vi "PicoScopeospaAdvancedTriggerSettings.vi"(0 "handle in":i16=16384, 2 "Trigger holdoff (Samples)":u64, 5 "error in":errorcluster, 6 "Trigger Conditions":T7={"Channel A"=1, "Channel B"=0, "Channel C"=0, "Channel D"=0, "Channel E"=0, "Channel F"=0, "Channel G"=0, "Channel H"=0, "Port 0"=0, "Port 1"=0, "Aux"=0, "PWQ"=0, "Condition Logic"=0} {"Port 1" items=["Don't Care", "True", "False"]; "Channel H" items=["Don't Care", "True", "False"]; "Channel G" items=["Don't Care", "True", "False"]; "Channel F" items=["Don't Care", "True", "False"]; "Channel E" items=["Don't Care", "True", "False"]; "PWQ" items=["Don't Care", "True", "False"]; "Aux" items=["Don't Care", "True", "False"]; "Port 0" items=["Don't Care", "True", "False"]; "Channel D" items=["Don't Care", "True", "False"]; "Channel C" items=["Don't Care", "True", "False"]; "Channel B" items=["Don't Care", "True", "False"]; "Channel A" items=["Don't Care", "True", "False"]; "Condition Logic" items=["AND", "OR", "XOR"]}, 7 "Pulse Width Qualifier Conditions":T1 {"Port 1" items=["Don't Care", "True", "False"]; "Channel H" items=["Don't Care", "True", "False"]; "Channel G" items=["Don't Care", "True", "False"]; "Channel F" items=["Don't Care", "True", "False"]; "Channel E" items=["Don't Care", "True", "False"]; "Aux" items=["Don't Care", "True", "False"]; "Port 0" items=["Don't Care", "True", "False"]; "Channel D" items=["Don't Care", "True", "False"]; "Channel C" items=["Don't Care", "True", "False"]; "Channel B" items=["Don't Care", "True", "False"]; "Channel A" items=["Don't Care", "True", "False"]; "Condition Logic" items=["AND", "OR", "XOR"]}, 8 "Channel Trigger Properties":T5={"Channel A Trigger Properties"={"thresholdUpper"=0, "thresholdUpperHysteresis"=1638, "thresholdLower"=0, "thresholdLowerHysteresis"=1638, "Threshold Mode"=0, "Direction"=2, "Available"=TRUE}, "Channel B Trigger Properties"={"thresholdUpper"=0, "thresholdUpperHysteresis"=1638, "thresholdLower"=0, "thresholdLowerHysteresis"=1638, "Threshold Mode"=0, "Direction"=2, "Available"=FALSE}, "Channel C Trigger Properties"={"thresholdUpper"=0, "thresholdUpperHysteresis"=1638, "thresholdLower"=0, "thresholdLowerHysteresis"=1638, "Threshold Mode"=0, "Direction"=2, "Available"=FALSE}, "Channel D Trigger Properties"={"thresholdUpper"=0, "thresholdUpperHysteresis"=1638, "thresholdLower"=0, "thresholdLowerHysteresis"=1638, "Threshold Mode"=0, "Direction"=2, "Available"=FALSE}, "Channel E Trigger Properties"={"thresholdUpper"=0, "thresholdUpperHysteresis"=0, "thresholdLower"=0, "thresholdLowerHysteresis"=0, "Threshold Mode"=0, "Direction"=2, "Available"=FALSE}, "Channel F Trigger Properties"={"thresholdUpper"=0, "thresholdUpperHysteresis"=0, "thresholdLower"=0, "thresholdLowerHysteresis"=0, "Threshold Mode"=0, "Direction"=2, "Available"=FALSE}, "Channel G Trigger Properties"={"thresholdUpper"=0, "thresholdUpperHysteresis"=0, "thresholdLower"=0, "thresholdLowerHysteresis"=0, "Threshold Mode"=0, "Direction"=2, "Available"=FALSE}, "Channel H Trigger Properties"={"thresholdUpper"=0, "thresholdUpperHysteresis"=0, "thresholdLower"=0, "thresholdLowerHysteresis"=0, "Threshold Mode"=0, "Direction"=2, "Available"=FALSE}} {"Channel H Trigger Properties"."Direction" items=["Above / Inside", "Below / Outside", "Rising / Enter", "Falling / Exit", "Rising or Falling / Enter or Exit", "Above Lower", "Below Lower", "Rising Lower", "Falling Lower", "Positive Runt", "Negative Runt"]; "Channel H Trigger Properties"."Threshold Mode" items=["Level", "Window"]; "Channel G Trigger Properties"."Direction" items=["Above / Inside", "Below / Outside", "Rising / Enter", "Falling / Exit", "Rising or Falling / Enter or Exit", "Above Lower", "Below Lower", "Rising Lower", "Falling Lower", "Positive Runt", "Negative Runt"]; "Channel G Trigger Properties"."Threshold Mode" items=["Level", "Window"]; "Channel F Trigger Properties"."Direction" items=["Above / Inside", "Below / Outside", "Rising / Enter", "Falling / Exit", "Rising or Falling / Enter or Exit", "Above Lower", "Below Lower", "Rising Lower", "Falling Lower", "Positive Runt", "Negative Runt"]; "Channel F Trigger Properties"."Threshold Mode" items=["Level", "Window"]; "Channel E Trigger Properties"."Direction" items=["Above / Inside", "Below / Outside", "Rising / Enter", "Falling / Exit", "Rising or Falling / Enter or Exit", "Above Lower", "Below Lower", "Rising Lower", "Falling Lower", "Positive Runt", "Negative Runt"]; "Channel E Trigger Properties"."Threshold Mode" items=["Level", "Window"]; "Channel D Trigger Properties"."Direction" items=["Above / Inside", "Below / Outside", "Rising / Enter", "Falling / Exit", "Rising or Falling / Enter or Exit", "Above Lower", "Below Lower", "Rising Lower", "Falling Lower", "Positive Runt", "Negative Runt"]; "Channel D Trigger Properties"."Threshold Mode" items=["Level", "Window"]; "Channel C Trigger Properties"."Direction" items=["Above / Inside", "Below / Outside", "Rising / Enter", "Falling / Exit", "Rising or Falling / Enter or Exit", "Above Lower", "Below Lower", "Rising Lower", "Falling Lower", "Positive Runt", "Negative Runt"]; "Channel C Trigger Properties"."Threshold Mode" items=["Level", "Window"]; "Channel B Trigger Properties"."Direction" items=["Above / Inside", "Below / Outside", "Rising / Enter", "Falling / Exit", "Rising or Falling / Enter or Exit", "Above Lower", "Below Lower", "Rising Lower", "Falling Lower", "Positive Runt", "Negative Runt"]; "Channel B Trigger Properties"."Threshold Mode" items=["Level", "Window"]; "Channel A Trigger Properties"."Direction" items=["Above / Inside", "Below / Outside", "Rising / Enter", "Falling / Exit", "Rising or Falling / Enter or Exit", "Above Lower", "Below Lower", "Rising Lower", "Falling Lower", "Positive Runt", "Negative Runt"]; "Channel A Trigger Properties"."Threshold Mode" items=["Level", "Window"]}, 9 "Pulse Width Qualifier Trigger Properties":T2={"Channel A Trigger Properties"={"Threshold Mode"=0, "Available"=TRUE, "Direction"=2}, "Channel B Trigger Properties"={"Threshold Mode"=0, "Available"=FALSE, "Direction"=2}, "Channel C Trigger Properties"={"Threshold Mode"=0, "Available"=FALSE, "Direction"=2}, "Channel D Trigger Properties"={"Threshold Mode"=0, "Available"=FALSE, "Direction"=2}, "Channel E Trigger Properties"={"Threshold Mode"=0, "Available"=FALSE, "Direction"=2}, "Channel F Trigger Properties"={"Threshold Mode"=0, "Available"=FALSE, "Direction"=2}, "Channel G Trigger Properties"={"Threshold Mode"=0, "Available"=FALSE, "Direction"=2}, "Channel H Trigger Properties"={"Threshold Mode"=0, "Available"=FALSE, "Direction"=2}, "Port 0 Trigger Properties"={"Threshold Mode"=0, "Available"=FALSE, "Direction"=2}, "Port 1 Trigger Properties"={"Threshold Mode"=0, "Available"=FALSE, "Direction"=2}} {"Port 1 Trigger Properties"."Direction" items=["Rising"=2, "Falling"=3, "Rising Lower"=7, "Above"=0, "Below"=1, "Rising or Falling"=4, "Falling Lower"=8, "Below Lower"=6, "Above Lower"=5]; "Port 1 Trigger Properties"."Threshold Mode" items=["Level", "Window"]; "Port 0 Trigger Properties"."Direction" items=["Rising"=2, "Falling"=3, "Rising Lower"=7, "Above"=0, "Below"=1, "Rising or Falling"=4, "Falling Lower"=8, "Below Lower"=6, "Above Lower"=5]; "Port 0 Trigger Properties"."Threshold Mode" items=["Level", "Window"]; "Channel H Trigger Properties"."Direction" items=["Rising"=2, "Falling"=3, "Rising Lower"=7, "Above"=0, "Below"=1, "Rising or Falling"=4, "Falling Lower"=8, "Below Lower"=6, "Above Lower"=5]; "Channel H Trigger Properties"."Threshold Mode" items=["Level", "Window"]; "Channel G Trigger Properties"."Direction" items=["Rising"=2, "Falling"=3, "Rising Lower"=7, "Above"=0, "Below"=1, "Rising or Falling"=4, "Falling Lower"=8, "Below Lower"=6, "Above Lower"=5]; "Channel G Trigger Properties"."Threshold Mode" items=["Level", "Window"]; "Channel F Trigger Properties"."Direction" items=["Rising"=2, "Falling"=3, "Rising Lower"=7, "Above"=0, "Below"=1, "Rising or Falling"=4, "Falling Lower"=8, "Below Lower"=6, "Above Lower"=5]; "Channel F Trigger Properties"."Threshold Mode" items=["Level", "Window"]; "Channel E Trigger Properties"."Direction" items=["Rising"=2, "Falling"=3, "Rising Lower"=7, "Above"=0, "Below"=1, "Rising or Falling"=4, "Falling Lower"=8, "Below Lower"=6, "Above Lower"=5]; "Channel E Trigger Properties"."Threshold Mode" items=["Level", "Window"]; "Channel D Trigger Properties"."Direction" items=["Rising"=2, "Falling"=3, "Rising Lower"=7, "Above"=0, "Below"=1, "Rising or Falling"=4, "Falling Lower"=8, "Below Lower"=6, "Above Lower"=5]; "Channel D Trigger Properties"."Threshold Mode" items=["Level", "Window"]; "Channel C Trigger Properties"."Direction" items=["Rising"=2, "Falling"=3, "Rising Lower"=7, "Above"=0, "Below"=1, "Rising or Falling"=4, "Falling Lower"=8, "Below Lower"=6, "Above Lower"=5]; "Channel C Trigger Properties"."Threshold Mode" items=["Level", "Window"]; "Channel B Trigger Properties"."Direction" items=["Rising"=2, "Falling"=3, "Rising Lower"=7, "Above"=0, "Below"=1, "Rising or Falling"=4, "Falling Lower"=8, "Below Lower"=6, "Above Lower"=5]; "Channel B Trigger Properties"."Threshold Mode" items=["Level", "Window"]; "Channel A Trigger Properties"."Direction" items=["Rising"=2, "Falling"=3, "Rising Lower"=7, "Above"=0, "Below"=1, "Rising or Falling"=4, "Falling Lower"=8, "Below Lower"=6, "Above Lower"=5]; "Channel A Trigger Properties"."Threshold Mode" items=["Level", "Window"]}, 10 "Digital Ports":T4 {"Digital Port  1"."Direction Channel 15" items=["Don't Care", "Low", "High", "Rising", "Falling"]; "Digital Port  1"."Direction Channel 14" items=["Don't Care", "Low", "High", "Rising", "Falling"]; "Digital Port  1"."Direction Channel 13" items=["Don't Care", "Low", "High", "Rising", "Falling"]; "Digital Port  1"."Direction Channel 12" items=["Don't Care", "Low", "High", "Rising", "Falling"]; "Digital Port  1"."Direction Channel 11" items=["Don't Care", "Low", "High", "Rising", "Falling"]; "Digital Port  1"."Direction Channel 10" items=["Don't Care", "Low", "High", "Rising", "Falling"]; "Digital Port  1"."Direction Channel 9" items=["Don't Care", "Low", "High", "Rising", "Falling"]; "Digital Port  1"."Direction Channel 8" items=["Don't Care", "Low", "High", "Rising", "Falling"]; "Digital Port  0"."Direction Channel 7" items=["Don't Care", "Low", "High", "Rising", "Falling"]; "Digital Port  0"."Direction Channel 6" items=["Don't Care", "Low", "High", "Rising", "Falling"]; "Digital Port  0"."Direction Channel 5" items=["Don't Care", "Low", "High", "Rising", "Falling"]; "Digital Port  0"."Direction Channel 4" items=["Don't Care", "Low", "High", "Rising", "Falling"]; "Digital Port  0"."Direction Channel 3" items=["Don't Care", "Low", "High", "Rising", "Falling"]; "Digital Port  0"."Direction Channel 2" items=["Don't Care", "Low", "High", "Rising", "Falling"]; "Digital Port  0"."Direction Channel 1" items=["Don't Care", "Low", "High", "Rising", "Falling"]; "Digital Port  0"."Direction Channel 0" items=["Don't Care", "Low", "High", "Rising", "Falling"]}, 11 "Pulse Width Qualifier Settings":T3 {"Pulse Width Type" items=["None", "Less Than", "Greater Than", "In Range", "Out of Range"]}, 12 "Auto Trigger (us)":u32=1000000 format="%.4p", 13 "Trigger Delay (samples)":u64) -> (14 "handle out":i16=16384, 19 "error out":errorcluster)   [LabVIEW 2010]
doc: "This VI is an interface for the advanced trigger features of the oscilloscope.\nA simple trigger can be set using PicoScopeXXXXSettings.vi, in which case it is not necessary to use this VI."
uses:
  psospa.dll
panel:
  in  "Addition Trigger Properties":T6={"Ext. Trigger Properties (DO NOT USE)"={"thresholdUpper"=0, "thresholdUpperHysteresis"=0, "thresholdLower"=0, "thresholdLowerHysteresis"=0, "Threshold Mode"=0, "Direction"=2, "Available"=FALSE}, "Aux. Trigger Properties"={"thresholdUpper"=0, "thresholdUpperHysteresis"=0, "thresholdLower"=0, "thresholdLowerHysteresis"=0, "Threshold Mode"=0, "Direction"=2, "Available"=FALSE}} {"Aux. Trigger Properties"."Direction" items=["Above / Inside", "Below / Outside", "Rising / Enter", "Falling / Exit", "Rising or Falling / Enter or Exit", "Above Lower", "Below Lower", "Rising Lower", "Falling Lower", "Positive Runt", "Negative Runt"]; "Aux. Trigger Properties"."Threshold Mode" items=["Level", "Window"]; "Ext. Trigger Properties (DO NOT USE)"."Direction" items=["Above / Inside", "Below / Outside", "Rising / Enter", "Falling / Exit", "Rising or Falling / Enter or Exit", "Above Lower", "Below Lower", "Rising Lower", "Falling Lower", "Positive Runt", "Negative Runt"]; "Ext. Trigger Properties (DO NOT USE)"."Threshold Mode" items=["Level", "Window"]}
  in  "SetTrigger Info Action XOR":bool=TRUE
  out "XOR Debug Array":u32[][](array[numeric])
  in  "SetTrigger Info Action OR":bool=TRUE
  # "For Condition Logic Suggested settings;\nFor AND, XOR logic-(parallel triggers)\nUse level-type triggers (Level or Inside/outside Window Triggers)\n\nFor OR logic- (single channel)\nUse edge types (e.g. rising, falling, entering window)"
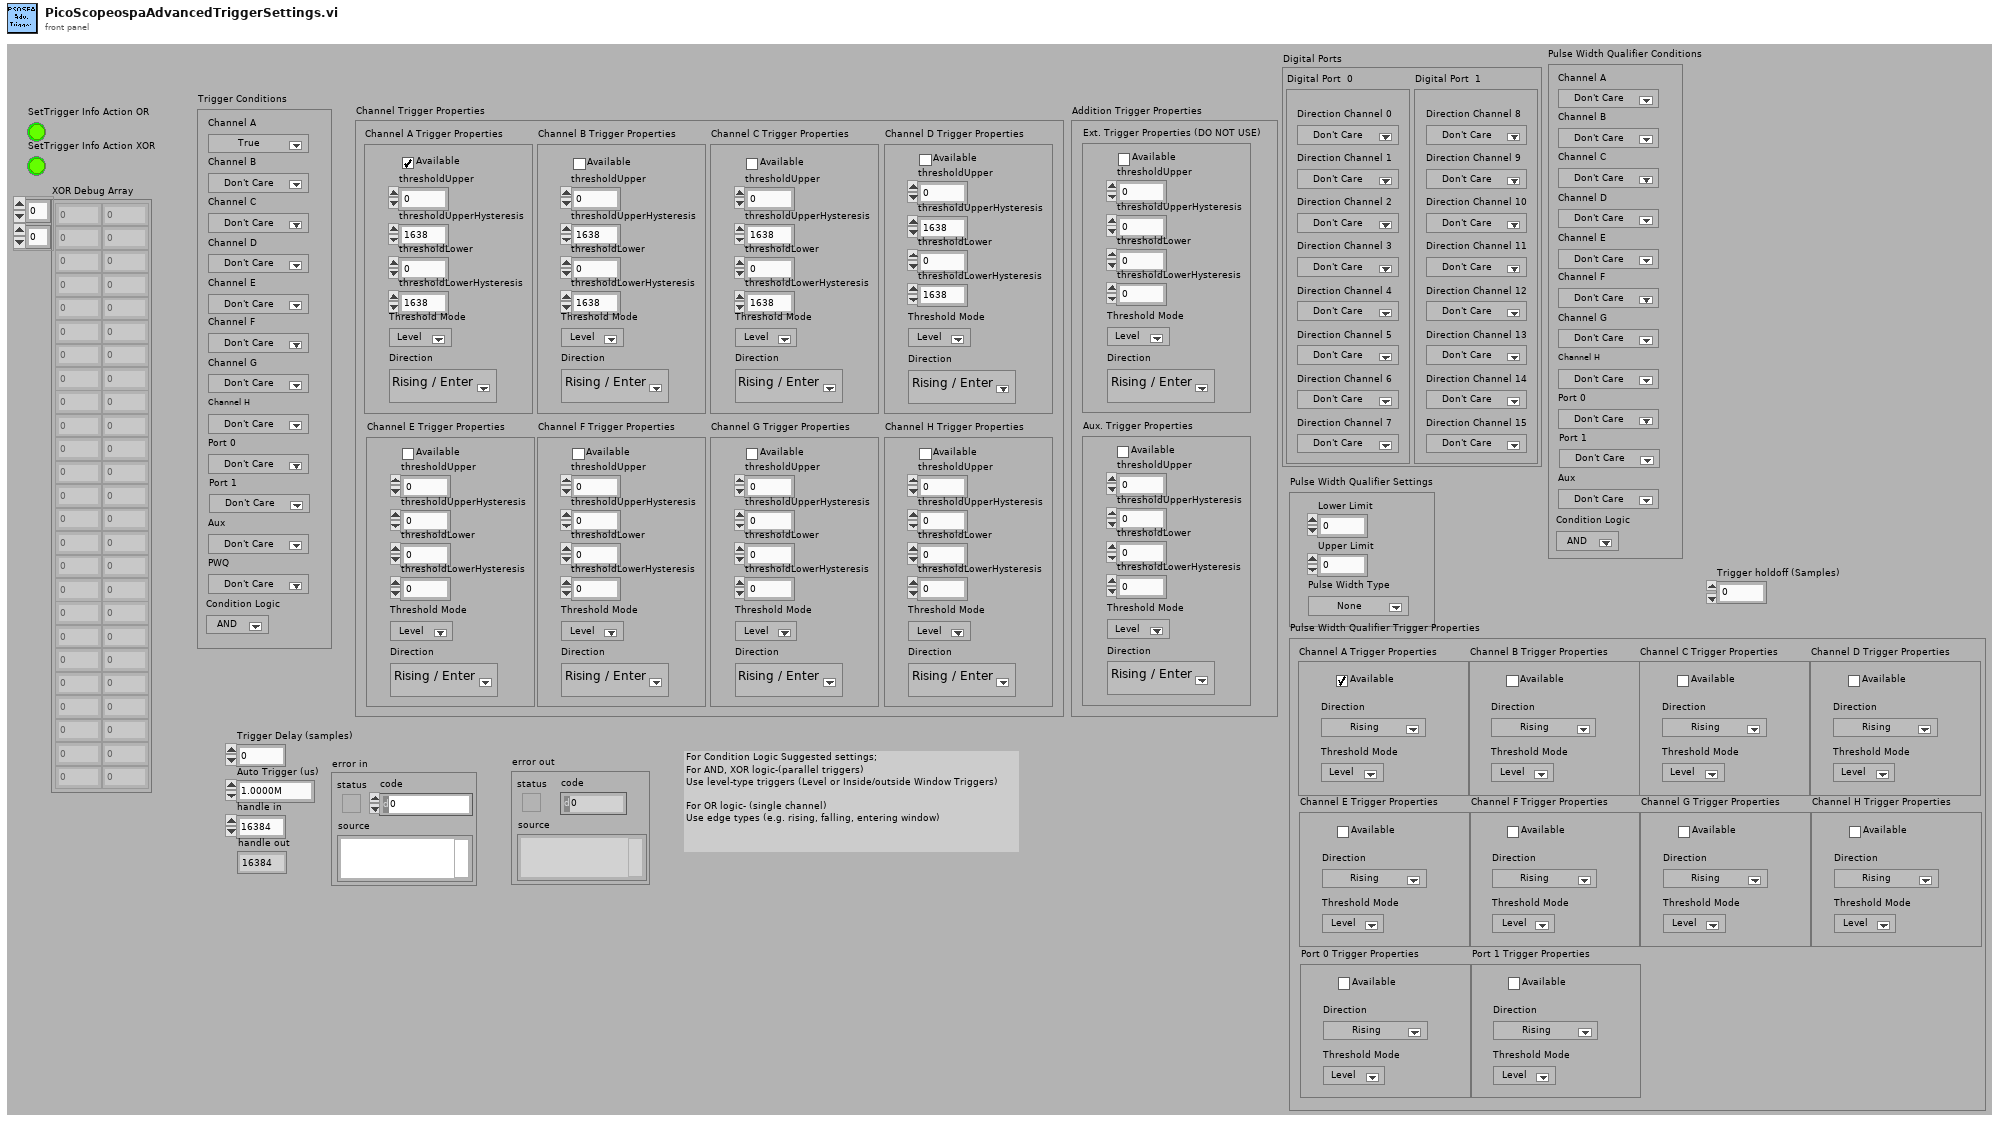
[diagram p1: front panel]
types:
  T1 = cluster{"Channel A":u16, "Channel B":u16, "Channel C":u16, "Channel D":u16, "Channel E":u16, "Channel F":u16, "Channel G":u16, "Channel H":u16, "Port 0":u16, "Port 1":u16, "Aux":u16, "Condition Logic":u16}
  T2 = cluster{"Channel A Trigger Properties":cluster{"Threshold Mode":i32, "Available":bool, "Direction":u32}, "Channel B Trigger Properties":cluster{"Threshold Mode":i32, "Available":bool, "Direction":u32}, "Channel C Trigger Properties":cluster{"Threshold Mode":i32, "Available":bool, "Direction":u32}, "Channel D Trigger Properties":cluster{"Threshold Mode":i32, "Available":bool, "Direction":u32}, "Channel E Trigger Properties":cluster{"Threshold Mode":i32, "Available":bool, "Direction":u32}, "Channel F Trigger Properties":cluster{"Threshold Mode":i32, "Available":bool, "Direction":u32}, "Channel G Trigger Properties":cluster{"Threshold Mode":i32, "Available":bool, "Direction":u32}, "Channel H Trigger Properties":cluster{"Threshold Mode":i32, "Available":bool, "Direction":u32}, "Port 0 Trigger Properties":cluster{"Threshold Mode":i32, "Available":bool, "Direction":u32}, "Port 1 Trigger Properties":cluster{"Threshold Mode":i32, "Available":bool, "Direction":u32}}
  T3 = cluster{"Lower Limit":u32, "Upper Limit":u32, "Pulse Width Type":u32}
  T4 = cluster{"Digital Port  0":cluster{"Direction Channel 0":u16, "Direction Channel 1":u16, "Direction Channel 2":u16, "Direction Channel 3":u16, "Direction Channel 4":u16, "Direction Channel 5":u16, "Direction Channel 6":u16, "Direction Channel 7":u16}, "Digital Port  1":cluster{"Direction Channel 8":u16, "Direction Channel 9":u16, "Direction Channel 10":u16, "Direction Channel 11":u16, "Direction Channel 12":u16, "Direction Channel 13":u16, "Direction Channel 14":u16, "Direction Channel 15":u16}}
  T5 = cluster{"Channel A Trigger Properties":cluster{"thresholdUpper":i16, "thresholdUpperHysteresis":u16, "thresholdLower":i16, "thresholdLowerHysteresis":u16, "Threshold Mode":i32, "Direction":i32, "Available":bool}, "Channel B Trigger Properties":cluster{"thresholdUpper":i16, "thresholdUpperHysteresis":u16, "thresholdLower":i16, "thresholdLowerHysteresis":u16, "Threshold Mode":i32, "Direction":i32, "Available":bool}, "Channel C Trigger Properties":cluster{"thresholdUpper":i16, "thresholdUpperHysteresis":u16, "thresholdLower":i16, "thresholdLowerHysteresis":u16, "Threshold Mode":i32, "Direction":i32, "Available":bool}, "Channel D Trigger Properties":cluster{"thresholdUpper":i16, "thresholdUpperHysteresis":u16, "thresholdLower":i16, "thresholdLowerHysteresis":u16, "Threshold Mode":i32, "Direction":i32, "Available":bool}, "Channel E Trigger Properties":cluster{"thresholdUpper":i16, "thresholdUpperHysteresis":u16, "thresholdLower":i16, "thresholdLowerHysteresis":u16, "Threshold Mode":i32, "Direction":i32, "Available":bool}, "Channel F Trigger Properties":cluster{"thresholdUpper":i16, "thresholdUpperHysteresis":u16, "thresholdLower":i16, "thresholdLowerHysteresis":u16, "Threshold Mode":i32, "Direction":i32, "Available":bool}, "Channel G Trigger Properties":cluster{"thresholdUpper":i16, "thresholdUpperHysteresis":u16, "thresholdLower":i16, "thresholdLowerHysteresis":u16, "Threshold Mode":i32, "Direction":i32, "Available":bool}, "Channel H Trigger Properties":cluster{"thresholdUpper":i16, "thresholdUpperHysteresis":u16, "thresholdLower":i16, "thresholdLowerHysteresis":u16, "Threshold Mode":i32, "Direction":i32, "Available":bool}}
  T6 = cluster{"Ext. Trigger Properties (DO NOT USE)":cluster{"thresholdUpper":i16, "thresholdUpperHysteresis":u16, "thresholdLower":i16, "thresholdLowerHysteresis":u16, "Threshold Mode":i32, "Direction":i32, "Available":bool}, "Aux. Trigger Properties":cluster{"thresholdUpper":i16, "thresholdUpperHysteresis":u16, "thresholdLower":i16, "thresholdLowerHysteresis":u16, "Threshold Mode":i32, "Direction":i32, "Available":bool}}
  T7 = cluster{"Channel A":u16, "Channel B":u16, "Channel C":u16, "Channel D":u16, "Channel E":u16, "Channel F":u16, "Channel G":u16, "Channel H":u16, "Port 0":u16, "Port 1":u16, "Aux":u16, "PWQ":u16, "Condition Logic":u16}
  T8 = cluster{"thresholdUpper":i16, "thresholdUpperHysteresis":u16, "thresholdLower":i16, "thresholdLowerHysteresis":u16, "Threshold Mode":i32, "Direction":i32, "Available":bool}[]
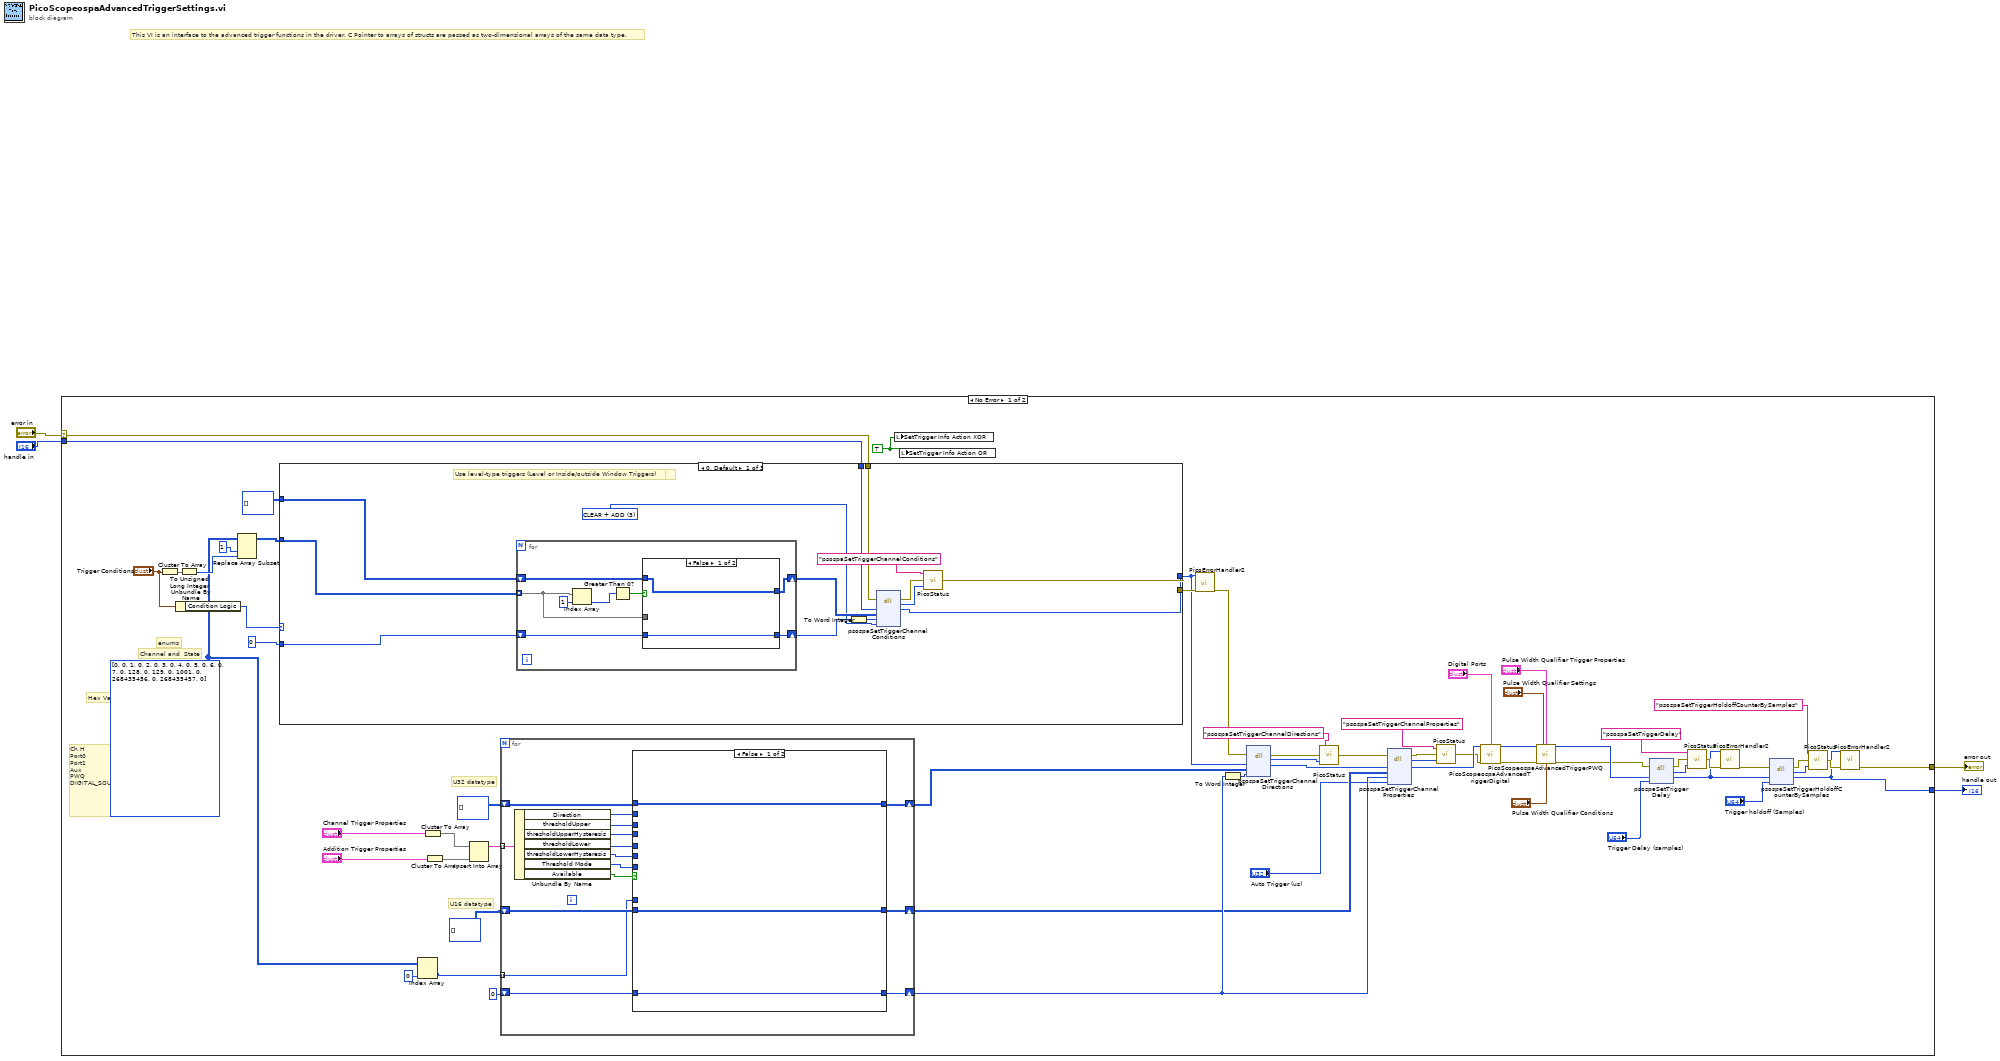
[diagram p0: block diagram]
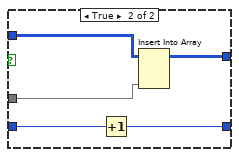
[diagram p2: hidden frame]
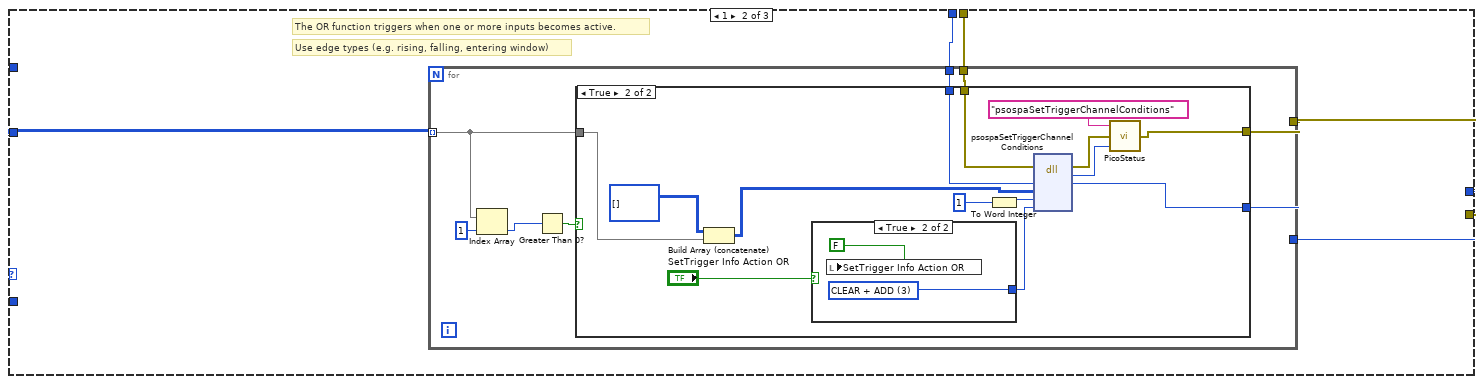
[diagram p3: hidden frame]
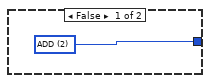
[diagram p5: hidden frame]
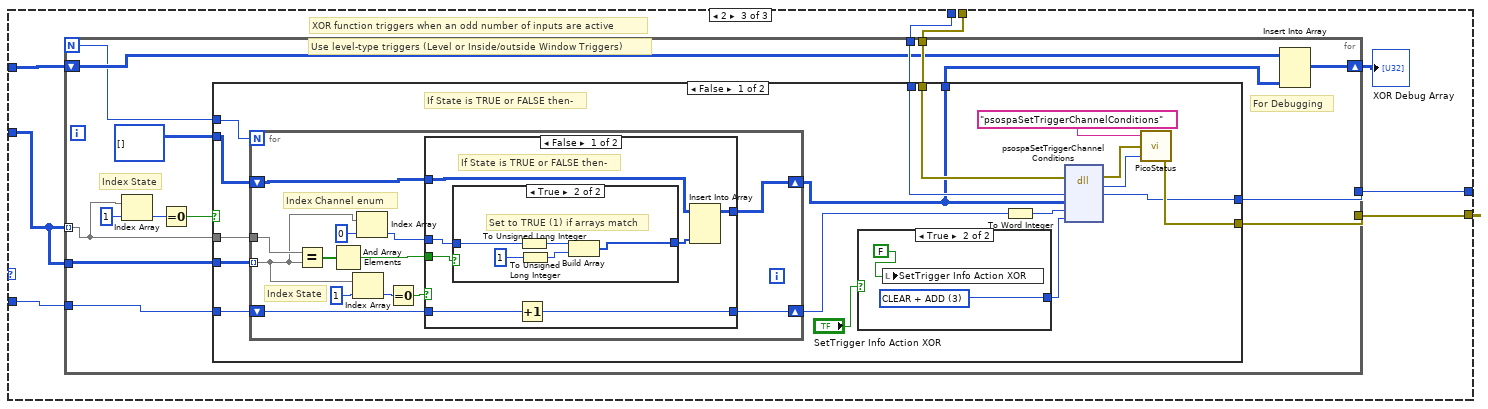
[diagram p6: hidden frame]
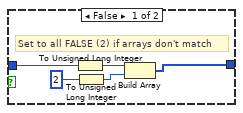
[diagram p7: hidden frame]
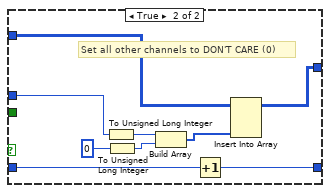
[diagram p8: hidden frame]
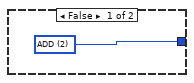
[diagram p9: hidden frame]
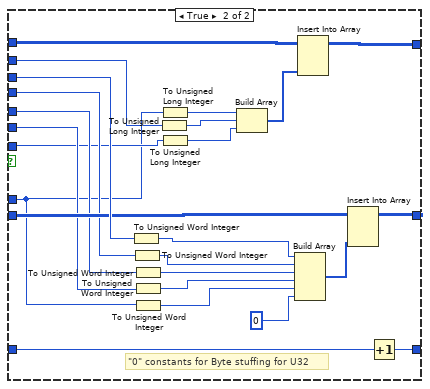
[diagram p11: hidden frame]
diagram:
  # "This VI is an interface to the advanced trigger functions in the driver. C Pointer to arrays of structs are passed as two-dimensional arrays of the same data type."
  n1 = case shown="No Error" "error in" {
    selector: "error in" -> [w36 w255]
    tunnel: "handle in" -> [w35 w256]
    tunnel: [w8 w256] -> w2
    tunnel: [w7 w255] -> w1
    frame No Error {
      w41 = TRUE ("Boolean")
      w26 = u32[][] [[0, 0], [1, 0], [2, 0], [3, 0], [4, 0], [5, 0], [6, 0], [7, 0], [128, 0], [129, 0], [1001, 0], [268435456, 0], [268435457, 0]]
      # "enums"
      # "Ch H\nPort0\nPort1\nAux\nPWQ\nDIGITAL_SOURCE"
      # "Channel and  State"
      # "Hex Values"
      # "U16 datatype"
      # "U32 datatype"
      n2 = Cluster To Array(cluster="Trigger Conditions") -> (array=w47:u16[])
      n3 = Unbundle By Name("Trigger Conditions") -> ("Condition Logic"=w28:u16)
      n4 = To Unsigned Long Integer(number=w47) -> (unsigned 32bit integer=w44:u32[])
      n5 = Replace Array Subset(array=w26, new element=w44, index (col)=1 ("disabled index (col)")) -> (w40:u32[][])  [unwired: 1 in]
      n6 = case shown="0, Default" w28 {
        tunnel: u32[][] [] -> [w80 _ w131]
        tunnel: i16 0 -> [w79 _ w128]
        tunnel: w36 -> [w73 w100 w135]
        tunnel: w35 -> [w72 w99 w134]
        tunnel: [w69 w98 w133] -> w38
        tunnel: [w68 w97 w132] -> w37
        tunnel: w40 -> [w67 w96 w129]
        frame 0, Default {
          w70 = u32 3 items=["CLEAR + ADD"=3, "CLEAR"=1, "ADD"=2] ("Condition Action")
          # "AND function requires both inputs to be active before it will trigger."
          # "Use level-type triggers (Level or Inside/outside Window Triggers)"
          n7 = for {
            shift-right: [w87] -> w75
            shift-left: w79 -> [w86]
            shift-right: [w85] -> w71
            shift-left: w80 -> [w88]
            tunnel: w67 -> [w83] mode=indexing
            n8 = Index Array(array=w83, index=1) -> (element=w82:u32)
            n9 = Greater Than 0?(x=w82) -> (x > 0?=w84:bool)
            n10 = case shown="False" w84 {
              tunnel: w88 -> [w90 w95]
              tunnel: [w90 w94] -> w85
              tunnel: [w89 w93] -> w87
              tunnel: w86 -> [w89 w92]
              tunnel: w83 -> [_ w91]
              frame False {
              }
              frame True {
                n11 = Increment(x=w92) -> (x+1=w93:i16)
                n12 = Insert Into Array(array=w95, new element=w91) -> (w94:u32[][])  [unwired: 2 in]
              }
            }
          }
          n13 = To Word Integer(number=w75) -> (16bit integer=w78:i16)
          n14 = dll-call lib="psospa.dll" fn="psospaSetTriggerChannelConditions" ("ps3000.dll:_ps3000_open_unit@0")(error in=w73, "handle"=w72, "conditions"=w71, "nConditions"=w78, "info"=w70) -> (error out=w77:errorcluster, "PICO_STATUS"=w76:u32, "handle"=w68:i16)  [unwired: 5 in, 1 out]
          n15 = call "PicoStatus.vi"("PICO STATUS"=w76, "error in"=w77, "source"="psospaSetTriggerChannelConditions") -> ("error out"=w69:errorcluster)
        }
        frame 1 {
          # "Use edge types (e.g. rising, falling, entering window)"
          # "The OR function triggers when one or more inputs becomes active."
          n16 = for {
            tunnel: w100 -> [w108]
            tunnel: w99 -> [w107]
            tunnel: [w106] -> w98
            tunnel: [w105] -> w97
            tunnel: w96 -> [w103] mode=indexing
            n17 = Index Array(array=w103, index=1) -> (element=w102:u32)
            n18 = Greater Than 0?(x=w102) -> (x > 0?=w101:bool)
            n19 = case shown="True" w101 {
              tunnel: w108 -> [w109 w120]
              tunnel: w107 -> [w110 w119]
              tunnel: [w109 w117] -> w106
              tunnel: [w110 w116] -> w105
              tunnel: w103 -> [_ w111]
              frame False {
              }
              frame True {
                n20 = Build Array (concatenate)(u32[][] [], w111) -> (w113:u32[][])
                n21 = case shown="True" "SetTrigger Info Action OR" {
                  tunnel: [w125 w127] -> w118
                  frame False {
                    w125 = u32 2 items=["CLEAR"=1, "ADD"=2, "CLEAR + ADD"=3] ("Condition Action")
                  }
                  frame True {
                    w127 = u32 3 items=["CLEAR"=1, "ADD"=2, "CLEAR + ADD"=3] ("Condition Action")
                    n22 = local write "SetTrigger Info Action OR"(FALSE ("Boolean")) -> ()
                  }
                }
                n23 = To Word Integer(number=i16 1) -> (16bit integer=w124:i16)
                n24 = dll-call lib="psospa.dll" fn="psospaSetTriggerChannelConditions" ("ps3000.dll:_ps3000_open_unit@0")(error in=w120, "handle"=w119, "conditions"=w113, "nConditions"=w124, "info"=w118) -> (error out=w123:errorcluster, "PICO_STATUS"=w122:u32, "handle"=w116:i16)  [unwired: 5 in, 1 out]
                n25 = call "PicoStatus.vi"("PICO STATUS"=w122, "error in"=w123, "source"="psospaSetTriggerChannelConditions") -> ("error out"=w117:errorcluster)
              }
            }
          }
        }
        frame 2 {
          # "Use level-type triggers (Level or Inside/outside Window Triggers)"
          # "XOR function triggers when an odd number of inputs are active"
          n26 = for {
            N -> [w143]
            tunnel: w135 -> [w150]
            tunnel: w134 -> [w149]
            tunnel: [w148] -> w133
            tunnel: [w147] -> w132
            shift-right: [w145] -> w130
            shift-left: w131 -> [w146]
            tunnel: w129 -> [w137] mode=indexing
            tunnel: w129 -> [w140]
            tunnel: w128 -> [w141]
            # "Index State"
            # "For Debugging"
            n27 = Index Array(array=w137, index=1) -> (element=w138:u32)
            n28 = Equal To 0?(x=w138) -> (x = 0?=w136:bool)
            n29 = case shown="False" w136 {
              tunnel: w150 -> [w167 w210]
              tunnel: w149 -> [w166 w211]
              tunnel: [w165 w210] -> w148
              tunnel: [w164 w211] -> w147
              tunnel: [w162 w212] -> w144
              tunnel: w143 -> [w161 _]
              tunnel: u32[][] [] -> [w160 w212]
              tunnel: w141 -> [w159 _]
              tunnel: w140 -> [w158 _]
              tunnel: w137 -> [w157 _]
              frame False {
                # "If State is TRUE or FALSE then-"
                n30 = for {
                  N: w161 -> [_]
                  shift-right: [w179] -> w163
                  shift-left: w159 -> [w180]
                  shift-right: [w168] -> w162
                  shift-left: w160 -> [w169]
                  tunnel: w157 -> [w176]
                  tunnel: w158 -> [w172] mode=indexing
                  # "Index State"
                  # "Index Channel enum"
                  n31 = Equal?(x=w176, y=w172) -> (x = y?=w170:bool[])
                  n32 = And Array Elements(Boolean array=w170) -> (logical AND=w175:bool)
                  n33 = Index Array(array=w172, index=1) -> (element=w173:u32)
                  n34 = Index Array(array=w172, index=0) -> (element=w177:u32)
                  n35 = Equal To 0?(x=w173) -> (x = 0?=w171:bool)
                  n36 = case shown="False" w171 {
                    tunnel: w180 -> [w187 w198]
                    tunnel: [w186 w199] -> w179
                    tunnel: w177 -> [w185 w202]
                    tunnel: w175 -> [w184 _]
                    tunnel: w169 -> [w183 w201]
                    tunnel: [w181 w200] -> w168
                    frame False {
                      # "If State is TRUE or FALSE then-"
                      n37 = case shown="True" w184 {
                        tunnel: [w192 w197] -> w182
                        tunnel: w185 -> [w191 w196]
                        frame False {
                          # "Set to all FALSE (2) if arrays don't match"
                          n38 = To Unsigned Long Integer(number=w191) -> (unsigned 32bit integer=w189:u32)
                          n39 = To Unsigned Long Integer(number=u32 2) -> (unsigned 32bit integer=w190:u32)
                          n40 = Build Array(w189, w190) -> (w192:u32[])
                        }
                        frame True {
                          # "Set to TRUE (1) if arrays match"
                          n41 = To Unsigned Long Integer(number=w196) -> (unsigned 32bit integer=w194:u32)
                          n42 = To Unsigned Long Integer(number=u32 1) -> (unsigned 32bit integer=w195:u32)
                          n43 = Build Array(w194, w195) -> (w197:u32[])
                        }
                      }
                      n44 = Increment(x=w187) -> (x+1=w186:i16)
                      n45 = Insert Into Array(array=w183, new element=w182) -> (w181:u32[][])  [unwired: 2 in]
                    }
                    frame True {
                      # "Set all other channels to DON'T CARE (0)"
                      n46 = To Unsigned Long Integer(number=w202) -> (unsigned 32bit integer=w204:u32)
                      n47 = To Unsigned Long Integer(number=u32 0) -> (unsigned 32bit integer=w205:u32)
                      n48 = Build Array(w204, w205) -> (w206:u32[])
                      n49 = Increment(x=w198) -> (x+1=w199:i16)
                      n50 = Insert Into Array(array=w201, new element=w206) -> (w200:u32[][])  [unwired: 2 in]
                    }
                  }
                }
                n51 = case shown="True" "SetTrigger Info Action XOR" {
                  tunnel: [w207 w209] -> w151
                  frame False {
                    w207 = u32 2 items=["CLEAR + ADD"=3, "CLEAR"=1, "ADD"=2] ("Condition Action")
                  }
                  frame True {
                    w209 = u32 3 items=["CLEAR + ADD"=3, "CLEAR"=1, "ADD"=2] ("Condition Action")
                    n52 = local write "SetTrigger Info Action XOR"(FALSE ("Boolean")) -> ()
                  }
                }
                n53 = To Word Integer(number=w163) -> (16bit integer=w156:i16)
                n54 = dll-call lib="psospa.dll" fn="psospaSetTriggerChannelConditions" ("ps3000.dll:_ps3000_open_unit@0")(error in=w167, "handle"=w166, "conditions"=w162, "nConditions"=w156, "info"=w151) -> (error out=w155:errorcluster, "PICO_STATUS"=w154:u32, "handle"=w164:i16)  [unwired: 5 in, 1 out]
                n55 = call "PicoStatus.vi"("PICO STATUS"=w154, "error in"=w155, "source"="psospaSetTriggerChannelConditions") -> ("error out"=w165:errorcluster)
              }
              frame True {
              }
            }
            n56 = Insert Into Array(array=w146, new element=w144) -> (w145:u32[][])  [unwired: 2 in]
          }
          "XOR Debug Array" <- w130
        }
      }
      n57 = Index Array(array=w26, index (col)=0 ("disabled index (col)")) -> (element=w25:u32[])  [unwired: 1 in]
      n58 = Cluster To Array(cluster="Channel Trigger Properties") -> (array=w32:T8)
      n59 = Cluster To Array(cluster="Addition Trigger Properties") -> (array=w30:T8)
      n60 = Insert Into Array(array=w32, new element=w30) -> (w31:T8)  [unwired: 1 in]
      n61 = for {
        tunnel: w31 -> [w214] mode=indexing
        shift-right: [w221] -> w49
        shift-left: i16 0 -> [w220]
        shift-right: [w218] -> w45
        shift-left: u16[][] [] -> [w219]
        shift-right: [w217] -> w46
        shift-left: u32[][] [] -> [w216]
        tunnel: w25 -> [w213] mode=indexing
        n62 = Unbundle By Name(w214) -> ("Direction"=w215:i32, "thresholdUpper"=w227:i16, "thresholdUpperHysteresis"=w226:u16, "thresholdLower"=w225:i16, "thresholdLowerHysteresis"=w224:u16, "Threshold Mode"=w223:i32, "Available"=w222:bool)
        n63 = case shown="False" w222 {
          tunnel: w227 -> [_ w254]
          tunnel: w226 -> [_ w240]
          tunnel: w225 -> [_ w239]
          tunnel: w224 -> [_ w238]
          tunnel: w223 -> [_ w235]
          tunnel: w213 -> [_ w232]
          tunnel: [w230 w253] -> w221
          tunnel: w220 -> [w230 w252]
          tunnel: [w229 w250] -> w218
          tunnel: w219 -> [w229 w249]
          tunnel: [w228 w248] -> w217
          tunnel: w216 -> [w228 w247]
          tunnel: w215 -> [_ w231]
          frame False {
          }
          frame True {
            # "\"0\" constants for Byte stuffing for U32"
            n64 = To Unsigned Word Integer(number=w254) -> (unsigned 16bit integer=w242:u16)
            n65 = To Unsigned Word Integer(number=w240) -> (unsigned 16bit integer=w241:u16)
            n66 = To Unsigned Word Integer(number=w239) -> (unsigned 16bit integer=w237:u16)
            n67 = To Unsigned Word Integer(number=w238) -> (unsigned 16bit integer=w243:u16)
            n68 = To Unsigned Word Integer(number=w232) -> (unsigned 16bit integer=w234:u16)
            n69 = To Unsigned Long Integer(number=w231) -> (unsigned 32bit integer=w245:u32)
            n70 = To Unsigned Long Integer(number=w232) -> (unsigned 32bit integer=w244:u32)
            n71 = To Unsigned Long Integer(number=w235) -> (unsigned 32bit integer=w236:u32)
            n72 = Build Array(w244, w245, w236) -> (w246:u32[])
            n73 = Build Array(w242, w241, w237, w243, w234, u16 0 ("element")) -> (w251:u16[])
            n74 = Insert Into Array(array=w247, new element=w246) -> (w248:u32[][])  [unwired: 2 in]
            n75 = Insert Into Array(array=w249, new element=w251) -> (w250:u16[][])  [unwired: 2 in]
            n76 = Increment(x=w252) -> (x+1=w253:i16)
          }
        }
      }
      n77 = local write "SetTrigger Info Action XOR"(w41) -> ()
      n78 = local write "SetTrigger Info Action OR"(w41) -> ()
      n79 = call "PicoErrorHandler2.vi"("error in (no error)"=w38, "handle In"=w37) -> ("error out"=w43:errorcluster)  [unwired: 9 in]
      n80 = To Word Integer(number=w49) -> (16bit integer=w50:i16)
      n81 = dll-call lib="psospa.dll" fn="psospaSetTriggerChannelDirections" ("ps3000.dll:_ps3000_open_unit@0")(error in=w43, "handle"=w37, "directions"=w46, "nDirections"=w50) -> (error out=w64:errorcluster, "PICO_STATUS"=w65:u32, "handle"=w66:i16)  [unwired: 4 in, 1 out]
      n82 = call "PicoStatus.vi"("PICO STATUS"=w65, "error in"=w64, "source"="psospaSetTriggerChannelDirections") -> ("error out"=w58:errorcluster)
      n83 = dll-call lib="psospa.dll" fn="psospaSetTriggerChannelProperties" ("ps3000.dll:_ps3000_open_unit@0")(error in=w58, "handle"=w66, "channelProperties"=w45, "nChannelProperties"=w49, "autoTriggerMicroSeconds"="Auto Trigger (us)") -> (error out=w62:errorcluster, "PICO_STATUS"=w63:u32, "handle"=w24:i16)  [unwired: 5 in, 1 out]
      n84 = call "PicoStatus.vi"("PICO STATUS"=w63, "error in"=w62, "source"="psospaSetTriggerChannelProperties") -> ("error out"=w23:errorcluster)
      n85 = call "PicoScopeospaAdvancedTriggerDigital.vi"("handle in"=w24, "Digital Ports"="Digital Ports", "error in"=w23) -> ("handle out"=w22:i16, "error out"=w21:errorcluster)  [unwired: 11 in]
      n86 = call "PicoScopeospaAdvancedTriggerPWQ.vi"("handle in"=w22, "Pulse Width Qualifier Settings"="Pulse Width Qualifier Settings", "Pulse Width Qualifier Trigger Properties"="Pulse Width Qualifier Trigger Properties", "error in"=w21, "Pulse Width Qualifier Conditions"="Pulse Width Qualifier Conditions") -> ("handle out"=w20:i16, "error out"=w19:errorcluster)  [unwired: 9 in]
      n87 = dll-call lib="psospa.dll" fn="psospaSetTriggerDelay" ("ps3000.dll:_ps3000_open_unit@0")(error in=w19, "handle"=w20, "delay"="Trigger Delay (samples)") -> (error out=w60:errorcluster, "PICO_STATUS"=w61:u32, "handle"=w9:i16)  [unwired: 3 in, 1 out]
      n88 = call "PicoStatus.vi"("PICO STATUS"=w61, "error in"=w60, "source"="psospaSetTriggerDelay") -> ("error out"=w59:errorcluster)
      n89 = call "PicoErrorHandler2.vi"("error in (no error)"=w59, "handle In"=w9) -> ("error out"=w10:errorcluster)  [unwired: 9 in]
      n90 = dll-call lib="psospa.dll" fn="psospaSetTriggerHoldoffCounterBySamples" ("ps3000.dll:_ps3000_open_unit@0")(error in=w10, "handle"=w9, "holdoffSamples"="Trigger holdoff (Samples)") -> (error out=w13:errorcluster, "PICO_STATUS"=w14:u32, "handle"=w8:i16)  [unwired: 3 in, 1 out]
      n91 = call "PicoStatus.vi"("PICO STATUS"=w14, "error in"=w13, "source"="psospaSetTriggerHoldoffCounterBySamples") -> ("error out"=w12:errorcluster)
      n92 = call "PicoErrorHandler2.vi"("error in (no error)"=w12, "handle In"=w8) -> ("error out"=w7:errorcluster)  [unwired: 9 in]
    }
    frame Error {
    }
  }
  "handle out" <- w2
  "error out" <- w1
